vi "SendActionPassOrFail.vi"(0 "session in":refnum<k35>, 7 "Action ToDo":string, 11 "error in":errorcluster) -> (4 "session out":refnum<k35>, 8 "Pass or Fail":string, 15 "error out":errorcluster)   [LabVIEW 2023]
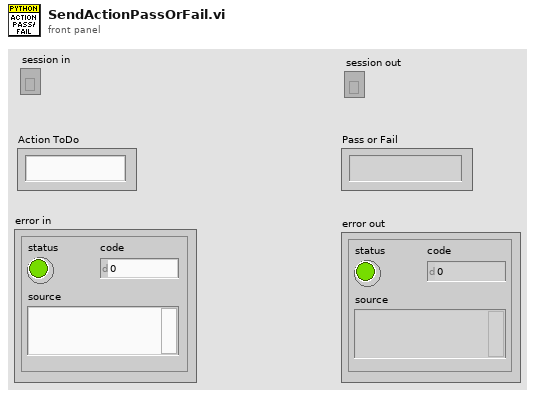
[diagram p1: front panel]
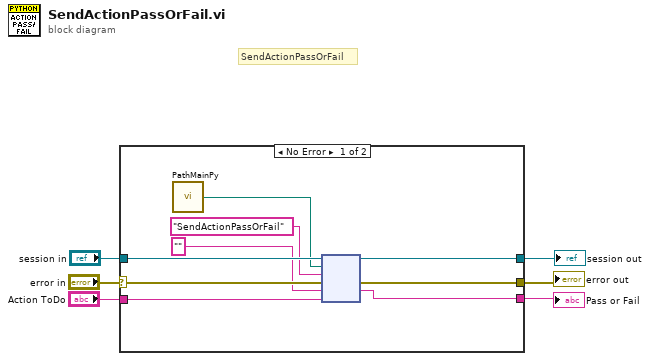
[diagram p0: block diagram]
diagram:
  # "SendActionPassOrFail"
  n1 = case shown="No Error" "error in" {
    selector: "error in" -> [w12 w16]
    tunnel: "session in" -> [w15 w17]
    tunnel: [w14 w17] -> w1
    tunnel: [w13 w16] -> w2
    tunnel: "Action ToDo" -> [w8 _]
    tunnel: [w7 _] -> w5
    frame No Error {
      n2 = call "PathMainPy.vi"() -> ("path"=w11:path)  [unwired: 15 in]
      n3 = node(w15, w11, "SendActionPassOrFail" ("function name"), w12, "" ("function name"), w8) -> (w14:refnum<k35>, w13:errorcluster, w7:string)  [unwired: 1 in, 2 out]
    }
    frame Error {
    }
  }
  "Pass or Fail" <- w5
  "error out" <- w2
  "session out" <- w1
